vi "Add item to ComboBox.vi"(8 "error in (no error)":errorcluster, 11 "Calling Actor in":refnum<class "Calling Actor.lvclass">) -> (0 "error out":errorcluster, 3 "Calling Actor out":refnum<class "Calling Actor.lvclass">)   [LabVIEW 2019, in "Calling Actor.lvlib" / "Calling Actor.lvclass"]
uses:
  Calling Actor.lvclass
  Calling Actor.lvclass/Calling Actor.ctl
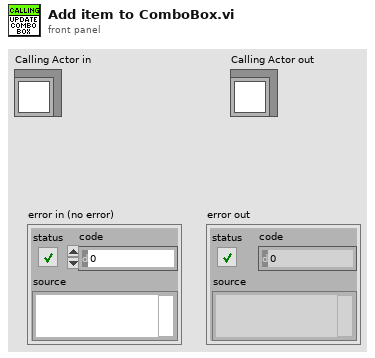
[diagram p1: front panel]
types:
  T1 = map{string, refnum<class "Message Enqueuer.lvclass">}
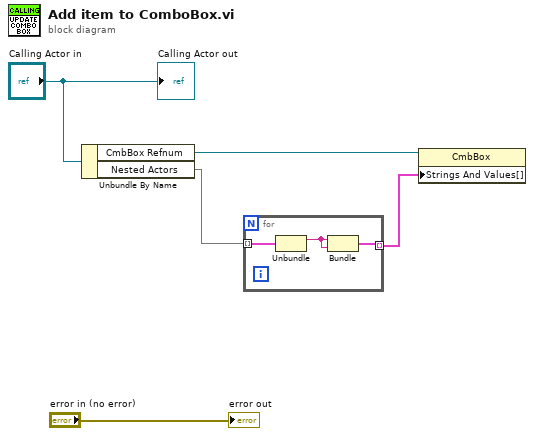
[diagram p0: block diagram]
diagram:
  n1 = Unbundle By Name("Calling Actor in") -> ("CmbBox Refnum"=w4:refnum<vi>, "Nested Actors"=w3:T1)
  n2 = for {
    tunnel: w3 -> [w8] mode=indexing
    tunnel: [w6] -> w2 mode=indexing
    n3 = Unbundle(w8) -> (w7:string)  [unwired: 1 out]
    n4 = Bundle(w7, w7) -> (w6:cluster{string, string})  [unwired: 1 in]
  }
  n5 = property class="CmbBox"(reference=w4, "Strings And Values[]"=w2) -> ()  [unwired: 1 in, 2 out]
  "Calling Actor out" <- "Calling Actor in"
  "error out" <- "error in (no error)"
